vi "Remove Viewer.vi"(8 "error in":errorcluster, 10 "viewer":T1, 11 "Data Server Thread in":refnum<class "Data Server Thread.lvclass">) -> (0 "error out":errorcluster, 3 "Data Server Thread out":refnum<class "Data Server Thread.lvclass">)   [LabVIEW 2021, in "DSF Core.lvlib" / "Data Server Thread.lvclass"]
uses:
  Data Server Thread.lvclass
  Viewer Data.ctl
  Buffer/Buffer.lvclass
  Status/Status Pointer.lvclass
  Data Server Thread.lvclass/Data Server Thread.ctl
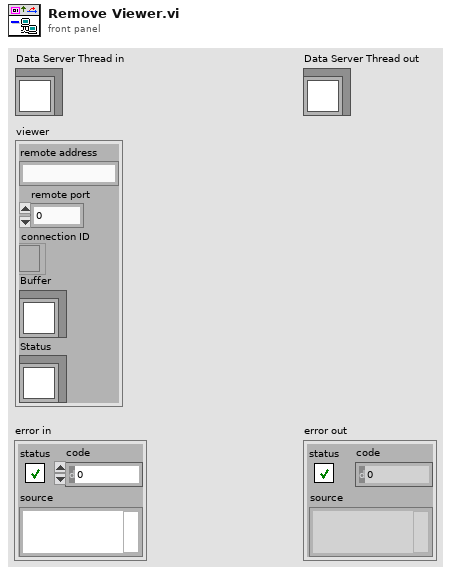
[diagram p1: front panel]
types:
  T1 = typedef "DSF Core.lvlib/Data Server Thread.lvclass/Viewer Data.ctl" = cluster{"remote address":string, "remote port":u16, "connection ID":refnum<k5>, "Buffer":refnum<class "Buffer.lvclass">, "Status":refnum<class "Status Pointer.lvclass">}
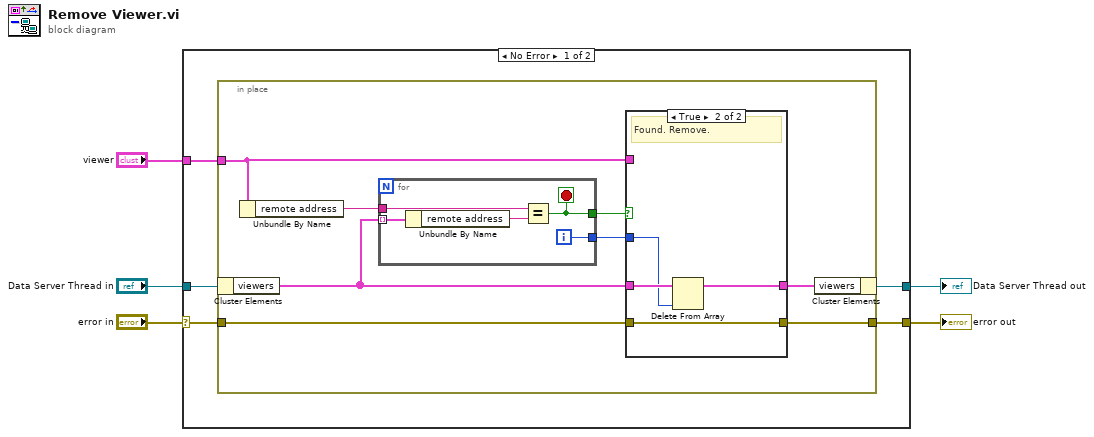
[diagram p0: block diagram]
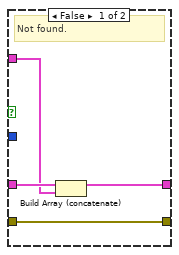
[diagram p2: hidden frame]
diagram:
  n1 = case shown="No Error" "error in" {
    selector: "error in" -> [w6 w33]
    tunnel: "Data Server Thread in" -> [w10 w32]
    tunnel: "viewer" -> [w9 _]
    tunnel: [w8 w33] -> w3
    tunnel: [w7 w32] -> w2
    frame No Error {
      n2 = in-place {
        in-place-border: w9 -> [w14]
        in-place-border: w6 -> [w12]
        in-place-border: [w11] -> w8
        n3 = in-place-cluster #1(w10) -> ("viewers"=w16:T1[])
        n4 = Unbundle By Name(w14) -> ("remote address"=w18:string)
        n5 = for {
          tunnel: w16 -> [w31] mode=indexing
          tunnel: w18 -> [w29]
          tunnel: [w28] -> w17
          tunnel: [w27] -> w13
          i -> [w27]
          stop <- w28 stop-if-true
          n6 = Unbundle By Name(w31) -> ("remote address"=w30:string)
          n7 = Equal?(x=w29, y=w30) -> (x = y?=w28:bool)
        }
        n8 = case shown="True" w17 {
          tunnel: w16 -> [w21 w26]
          tunnel: [w22 w24] -> w15
          tunnel: w14 -> [w20 _]
          tunnel: w13 -> [_ w23]
          tunnel: w12 -> [w19 w25]
          tunnel: [w19 w25] -> w11
          frame False {
            # "Not found."
            n9 = Build Array (concatenate)(w21, w20) -> (w22:T1[])
          }
          frame True {
            # "Found. Remove."
            n10 = Delete From Array(array=w26, index=w23) -> (array with subset deleted=w24:T1[])  [unwired: 1 in, 1 out]
          }
        }
        n11 = in-place-cluster #1("viewers"=w15) -> (w7:refnum<class "Data Server Thread.lvclass">)
      }
    }
    frame Error {
    }
  }
  "error out" <- w3
  "Data Server Thread out" <- w2
